vi "read_occupancy_OLD.vi"() -> ()   [LabVIEW 2011]
uses:
  Dependencies/global.vi
panel:
  out "Events":u32[][](array[numeric])
  out "Reset":bool=TRUE
  in  "Reset to Number:":dbl
  in  "Reset Counter":bool
  in  "Reset at:":string="00:00:00"
  out "Current Time":string
  out "Occupancy":T1(graph)
  out "element":string
  out "Deque error":errorcluster
  out "DataSocket error":errorcluster
  out "# Sent Data":u64
  out "The number of people inside A:225:":dbl
  in  "Initial number of people inside A:225:":dbl
  out "Estimated events":dbl[](array[numeric])
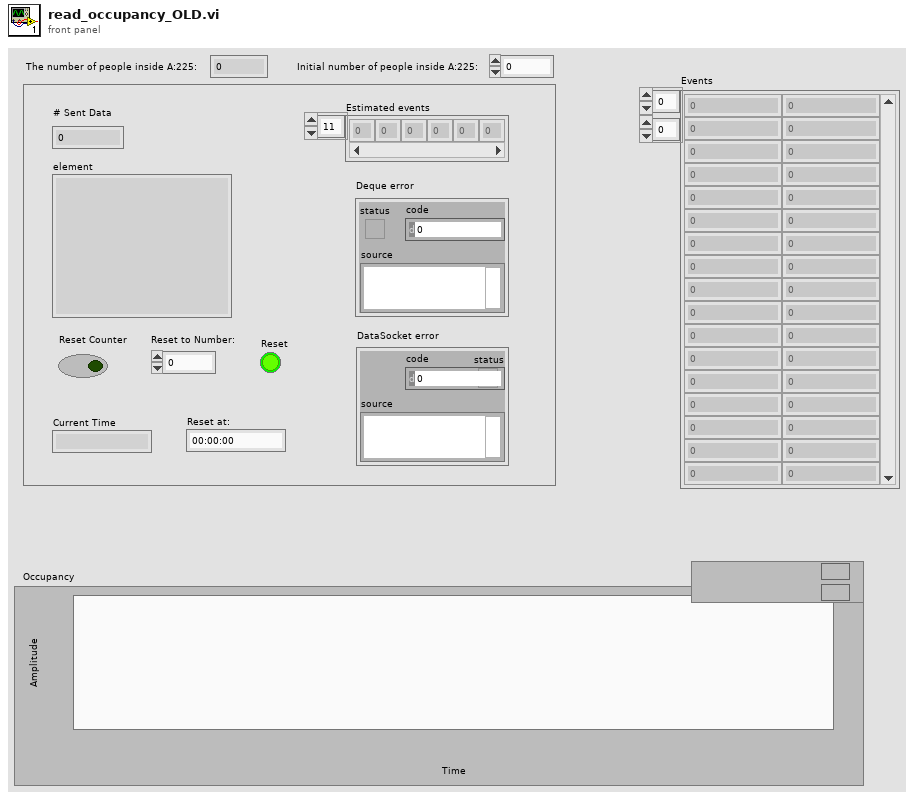
[diagram p1: front panel]
types:
  T1 = cluster{"The number of people inside A:225:":dbl, "Estimated Occupancy":dbl}
  T2 = enum16{"Read", "Write", "ReadWrite", "BufferedRead", "BufferedReadWrite"}
  T3 = cluster{"The number of people inside A:225:":dbl, "Estimated Occupancy":dbl}[]
  T4 = typedef "imagedata.ctl" = cluster{"image type":i32, "image depth":i32, "image":u8[], "mask":u8[], "colors":u32[], "Rectangle":cluster{"left":i16, "top":i16, "right":i16, "bottom":i16}}
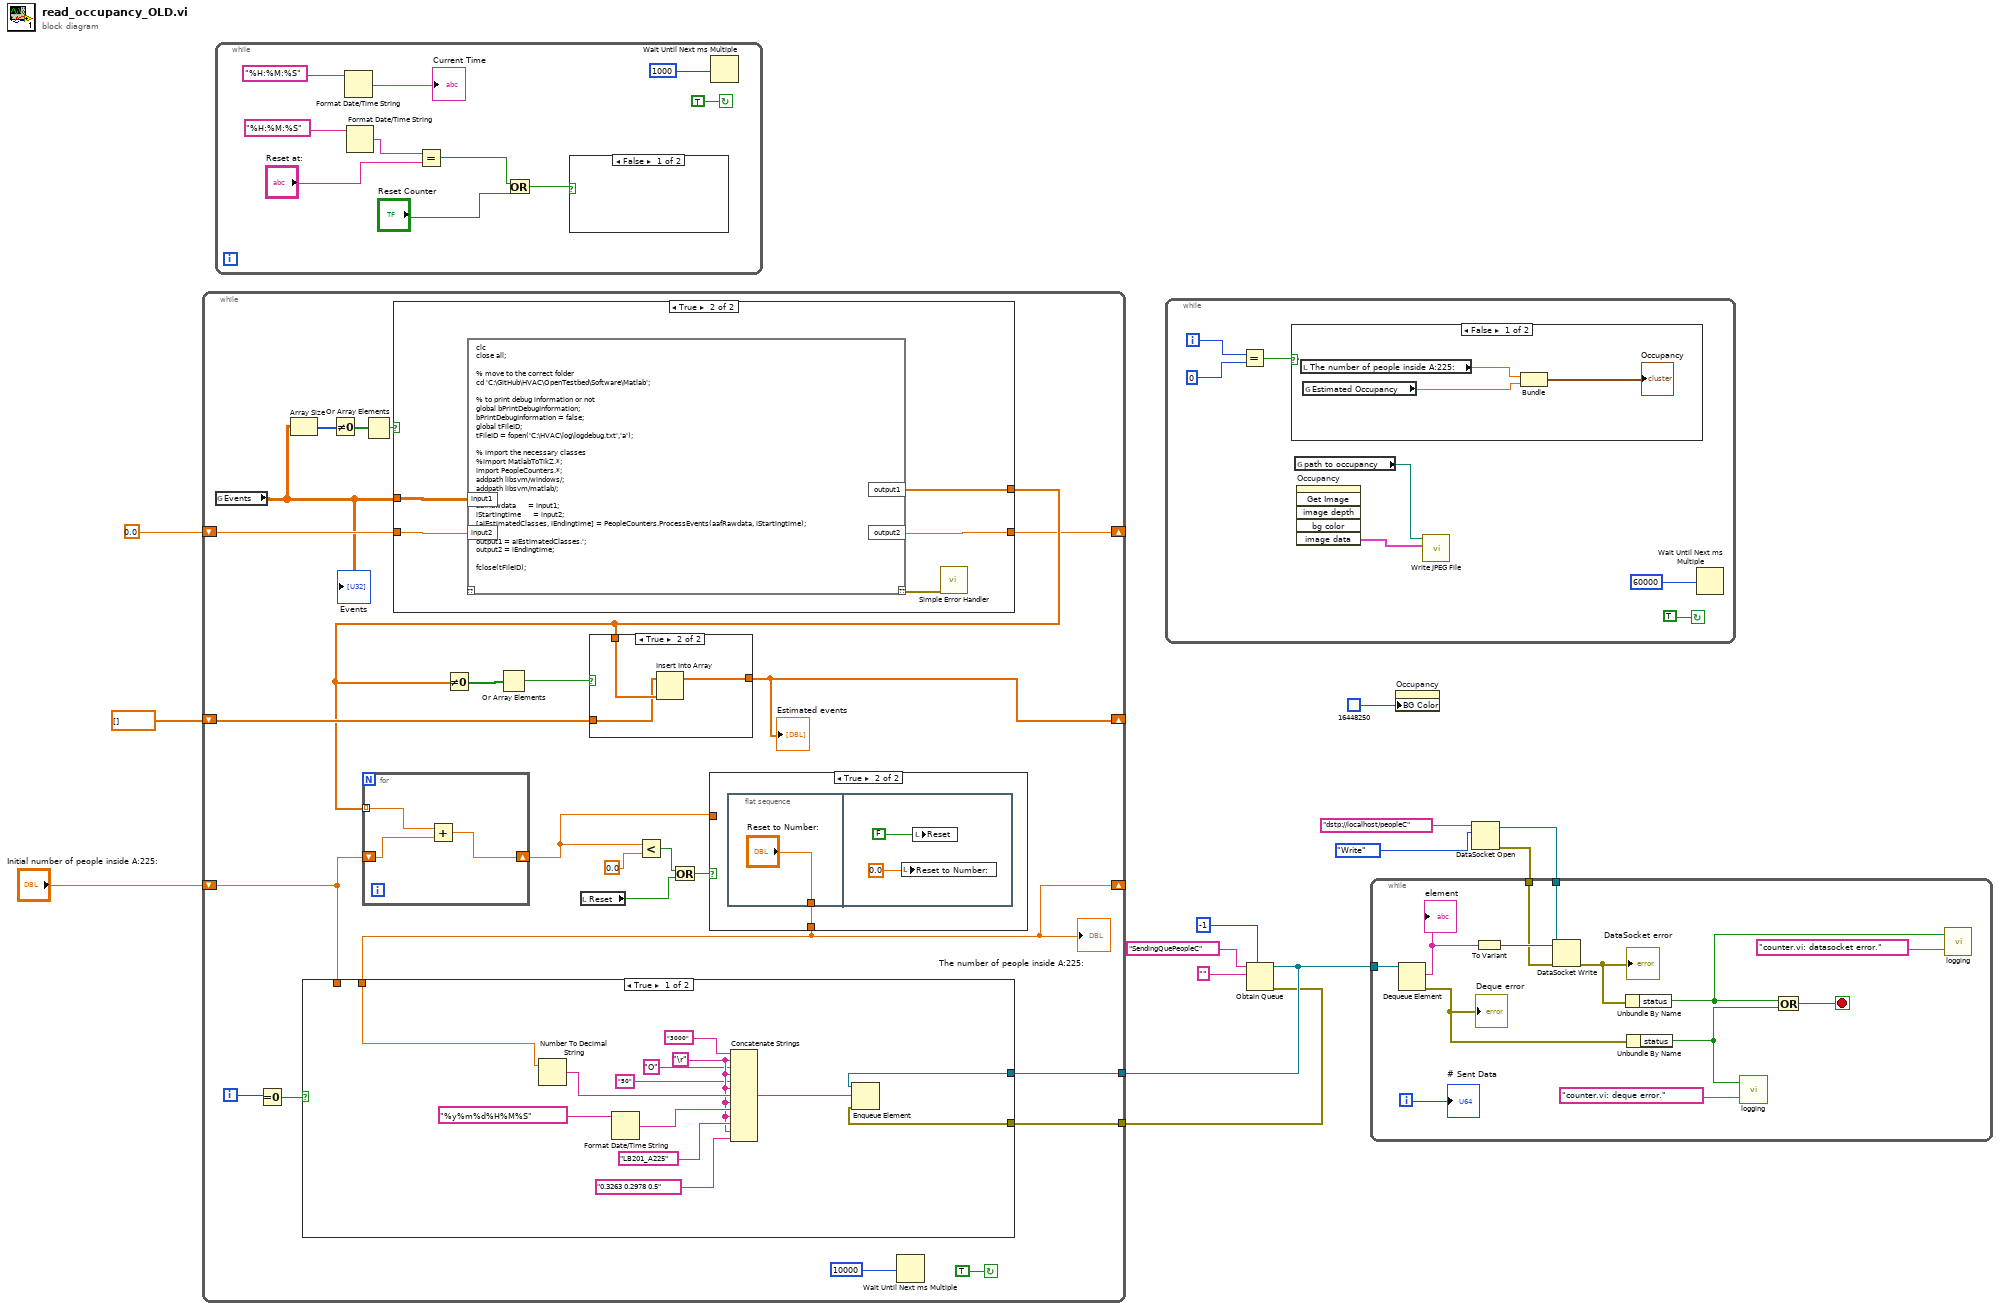
[diagram p0: block diagram]
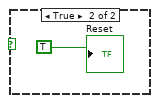
[diagram p2: hidden frame]
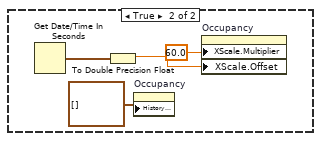
[diagram p3: hidden frame]
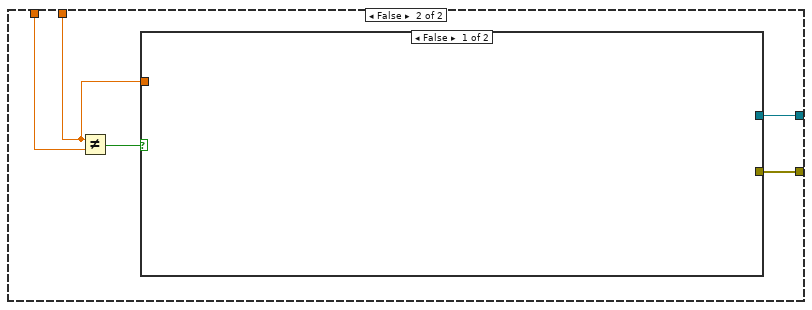
[diagram p5: hidden frame]
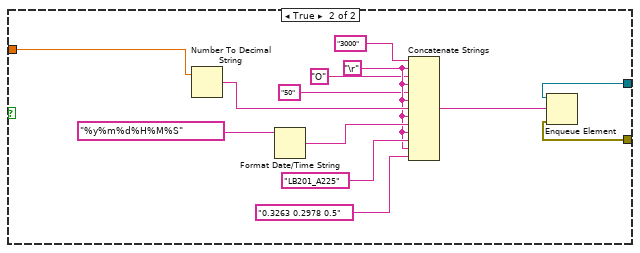
[diagram p6: hidden frame]
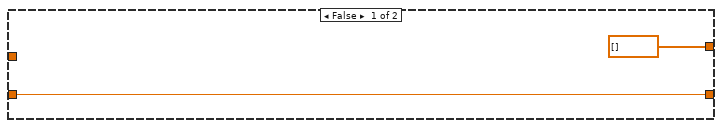
[diagram p8: hidden frame]
diagram:
  n1 = while {
    stop <- TRUE continue-if-true
    n2 = Format Date/Time String(time format string (%c)="%H:%M:%S") -> (date/time string=→"Current Time":string)  [unwired: 2 in]
    n3 = Format Date/Time String(time format string (%c)="%H:%M:%S") -> (date/time string=w20:string)  [unwired: 2 in]
    n4 = Equal?(x=w20, y="Reset at:") -> (x = y?=w16:bool)
    n5 = Or(x=w16, y="Reset Counter") -> (x .or. y?=w15:bool)
    n6 = case shown="False" w15 {
      frame False {
      }
      frame True {
        "Reset" <- TRUE ("Reset Counter")
      }
    }
    n7 = Wait Until Next ms Multiple(millisecond multiple=u32 1000 ("milliseconds to wait")) -> ()  [unwired: 1 out]
  }
  n8 = while {
    i -> [w28]
    stop <- TRUE continue-if-true
    n9 = Equal?(x=w28, y=i16 0) -> (x = y?=w30:bool)
    n10 = case shown="False" w30 {
      frame False {
        n11 = local read "The number of people inside A:225:"() -> (w32:dbl)
        n12 = global read "global.vi" "Estimated Occupancy"() -> (w34:dbl)
        n13 = Bundle("The number of people inside A:225:"=w32, "Estimated Occupancy"=w34) -> (→"Occupancy":T1)  [unwired: 1 in]
      }
      frame True {
        n14 = Get Date/Time In Seconds() -> (seconds since 1Jan1904=w38:timestamp)
        n15 = To Double Precision Float(number=w38) -> (double precision float=w37:dbl)
        n16 = property on="Occupancy" class="WFChart (strict)"("History Data"=T3 []) -> ()  [unwired: 2 in, 2 out]
        n17 = property on="Occupancy" class="WFChart (strict)"("XScale.Multiplier"=60.0 ("X Scale.Offset and Multiplier:Multiplier"), "XScale.Offset"=w37) -> ()  [unwired: 2 in, 2 out]
      }
    }
    n18 = global read "global.vi" "path to occupancy"() -> (w26:path)
    n19 = invoke on="Occupancy" class="WFChart (strict)" method="Get Image"() -> ("image data"=w27:T4)  [unwired: 6 in, 5 out]
    n20 = call <vilib>:"Write JPEG File.vi"("image data"=w27, "path to JPEG file"=w26) -> ()  [unwired: 8 in, 2 out]
    n21 = Wait Until Next ms Multiple(millisecond multiple=u32 60000 ("milliseconds to wait")) -> ()  [unwired: 1 out]
  }
  n22 = Obtain Queue(max queue size (-1, unlimited)=-1, name (unnamed)="SendingQuePeopleC", element data type="") -> (queue out=w6:refnum<queue>, error out=w5:errorcluster)  [unwired: 2 in, 1 out]
  n23 = while {
    shift-right: [w52] -> _
    shift-left: 0.0 ("Real Matrix Element") -> [w61]
    shift-right: [w53] -> _
    shift-left: dbl[] [] -> [w60]
    shift-right: [w39] -> _
    shift-left: "Initial number of people inside A:225:" -> [w50]
    tunnel: w6 -> [w49]
    tunnel: w5 -> [w48]
    i -> [w47]
    stop <- TRUE continue-if-true
    n24 = global read "global.vi" "Events"() -> (w45:dbl[][])
    "Events" <- w45
    n25 = Equal To 0?(x=w47) -> (x = 0?=w46:bool)
    n26 = Array Size(array=w45) -> (size(s)=w59:i32[])
    n27 = Not Equal To 0?(x=w59) -> (x != 0?=w58:bool[])
    n28 = Or Array Elements(Boolean array=w58) -> (logical OR=w57:bool)
    n29 = case shown="True" w57 {
      tunnel: w61 -> [w106 w112]
      tunnel: [w106 w111] -> w52
      tunnel: [dbl[] [] w110] -> w54
      tunnel: w45 -> [_ w109]
      frame False {
      }
      frame True {
        n30 = script code="clc\nclose all;\n\n% move to the correct folder\ncd 'C:\\GitHub\\HVAC\\OpenTestbed\\Software\\Matlab';\n\n% to print debug information or not\nglobal bPrintDebugInformation;\nbPrintDebugInformation = false;\nglobal tFileID;\ntFileID = fopen('C:\\HVAC\\log\\logdebug.txt','a');\n\n% import the necessary classes\n%import MatlabToTikZ.*;\nimport PeopleCounters.*;\naddpath libsvm/windows/;\naddpath libsvm/matlab/;\n\naafRawdata      = input1;\niStartingtime      = input2;\n[aiEstimatedClasses, iEndingtime] = PeopleCounters.ProcessEvents(aafRawdata, iStartingtime);\n\noutput1 = aiEstimatedClasses.';\noutput2 = iEndingtime;\n\nfclose(tFileID);"("input1"=w109, "input2"=w112) -> ("??"=w108:errorcluster, "output1"=w110:dbl[], "output2"=w111:dbl)  [unwired: 1 in]
        n31 = call <vilib>:"Simple Error Handler.vi"("error in (no error)"=w108) -> ()  [unwired: 4 in, 5 out]
      }
    }
    n32 = for {
      tunnel: w54 -> [w101] mode=indexing
      shift-right: [w99] -> w43
      shift-left: w50 -> [w100]
      n33 = Add(x=w101, y=w100) -> (x+y=w99:dbl)
    }
    n34 = Not Equal To 0?(x=w54) -> (x != 0?=w56:bool[])
    n35 = Or Array Elements(Boolean array=w56) -> (logical OR=w55:bool)
    n36 = local read "Reset"() -> (w40:bool)
    n37 = case shown="True" w55 {
      tunnel: w54 -> [_ w105]
      tunnel: w60 -> [w102 w104]
      tunnel: [w102 w103] -> w53
      frame False {
      }
      frame True {
        n38 = Insert Into Array(array=w104, new element=w105) -> (w103:dbl[])  [unwired: 1 in]
      }
    }
    "Estimated events" <- w53
    n39 = Less?(x=w43, y=0.0) -> (x < y?=w42:bool)
    n40 = Or(x=w42, y=w40) -> (x .or. y?=w41:bool)
    n41 = case shown="True" w41 {
      tunnel: w43 -> [w63 _]
      tunnel: [w63 w64] -> w39
      frame False {
      }
      frame True {
        n42 = flat-sequence {
          tunnel: ["Reset to Number:"] -> w64
          frame #0 {
          }
          frame #1 {
            n43 = local write "Reset to Number:"(0.0 ("Reset to Number:")) -> ()
            n44 = local write "Reset"(FALSE ("Reset")) -> ()
          }
        }
      }
    }
    "The number of people inside A:225:" <- w39
    n45 = case shown="True" w46 {
      tunnel: w39 -> [w68 w84]
      tunnel: w50 -> [_ w83]
      tunnel: w49 -> [w70 w82]
      tunnel: w48 -> [w69 w81]
      frame True {
        w75 = "\r"
        n46 = Number To Decimal String(number=w68) -> (decimal integer string=w79:string)  [unwired: 1 in]
        n47 = Format Date/Time String(time format string (%c)="%y%m%d%H%M%S") -> (date/time string=w77:string)  [unwired: 2 in]
        n48 = Concatenate Strings("3000" ("string"), w75, "O" ("string"), w75, "50" ("string"), w75, w79, w75, w77, w75, "LB201_A225", w75, "0.3263 0.2978 0.5" ("string")) -> (w71:string)
        n49 = Enqueue Element(queue=w70, element=w71, error in (no error)=w69) -> ()  [unwired: 1 in, 3 out]
      }
      frame False {
        n50 = Not Equal?(x=w84, y=w83) -> (x != y?=w85:bool)
        n51 = case shown="False" w85 {
          tunnel: w82 -> [_ w88]
          tunnel: w81 -> [_ w87]
          tunnel: w84 -> [_ w86]
          frame False {
          }
          frame True {
            w93 = "\r"
            n52 = Number To Decimal String(number=w86) -> (decimal integer string=w97:string)  [unwired: 1 in]
            n53 = Format Date/Time String(time format string (%c)="%y%m%d%H%M%S") -> (date/time string=w95:string)  [unwired: 2 in]
            n54 = Concatenate Strings("3000" ("string"), w93, "O" ("string"), w93, "50" ("string"), w93, w97, w93, w95, w93, "LB201_A225", w93, "0.3263 0.2978 0.5" ("string")) -> (w89:string)
            n55 = Enqueue Element(queue=w88, element=w89, error in (no error)=w87) -> ()  [unwired: 1 in, 3 out]
          }
        }
      }
    }
    n56 = Wait Until Next ms Multiple(millisecond multiple=u32 10000 ("milliseconds to wait")) -> ()  [unwired: 1 out]
  }
  n57 = property on="Occupancy" class="WFChart (strict)"("BG Color"=u32 16448250) -> ()  [unwired: 2 in, 2 out]
  n58 = DataSocket Open(10:T2."Write" ("mode"), 11:"dstp://localhost/peopleC" ("URL 3")) -> (0:w13:errorcluster, 3:w12:refnum<k13>)  [unwired: 2 in]
  n59 = while {
    tunnel: w6 -> [w125]
    tunnel: w12 -> [w124]
    tunnel: w13 -> [w120]
    i -> [w118]
    stop <- w119 stop-if-true
    n60 = Dequeue Element(queue=w125) -> (element=w113:string, error out=w122:errorcluster)  [unwired: 2 in, 2 out]
    "Deque error" <- w122
    "element" <- w113
    n61 = To Variant(anything=w113) -> (Variant=w123:variant)
    n62 = DataSocket Write(8:w120, 10:w123, 11:w124) -> (0:w121:errorcluster)  [unwired: 3 out]
    "DataSocket error" <- w121
    n63 = Unbundle By Name(w121) -> ("status"=w114:bool)
    n64 = Unbundle By Name(w122) -> ("status"=w116:bool)
    n65 = call "logging.vi"("data"="counter.vi: deque error.", "Boolean"=w116) -> ()  [unwired: 1 in]
    n66 = Compound Arithmetic op=OR(w114, w116) -> (w119:bool)
    n67 = call "logging.vi"("data"="counter.vi: datasocket error.", "Boolean"=w114) -> ()  [unwired: 1 in]
    "# Sent Data" <- w118
  }
